vi "MonitorAlert.vi"(8 "error in (no error)":errorcluster, 10 "Str Refnum":refnum<vi>, 11 "Handle":i32) -> (0 "error out":errorcluster)   [LabVIEW 2016]
uses:
  kernel32.dll
panel:
  out "Array":u8[](array[numeric])
  out "Return":u8
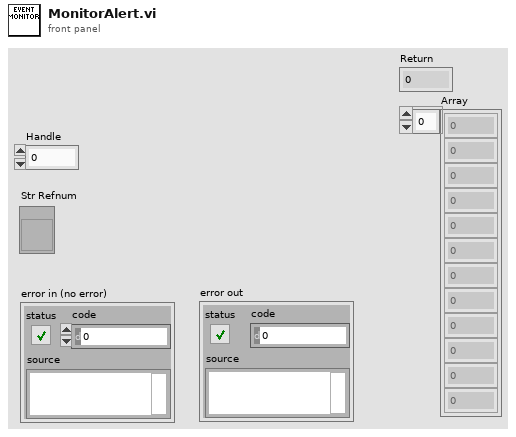
[diagram p1: front panel]
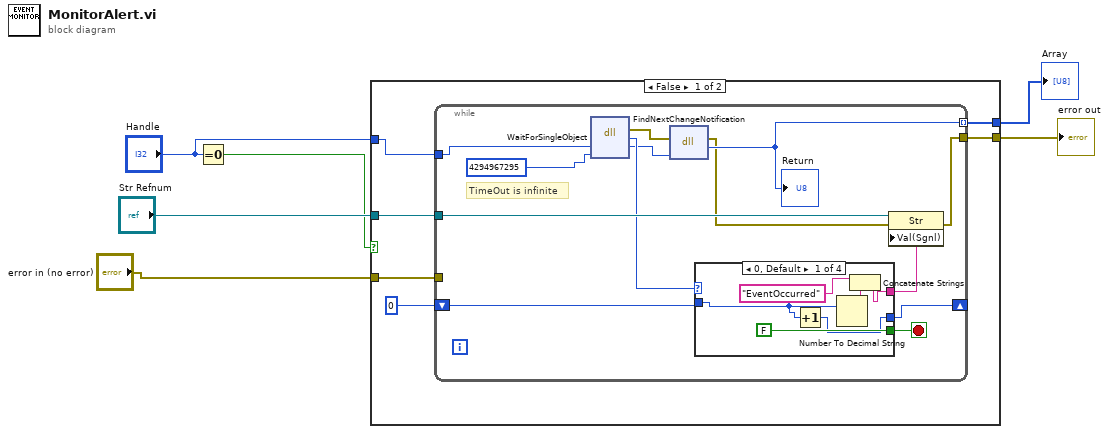
[diagram p0: block diagram]
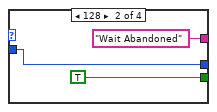
[diagram p2: hidden frame]
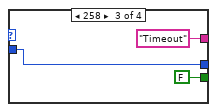
[diagram p3: hidden frame]
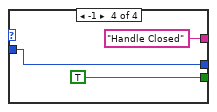
[diagram p4: hidden frame]
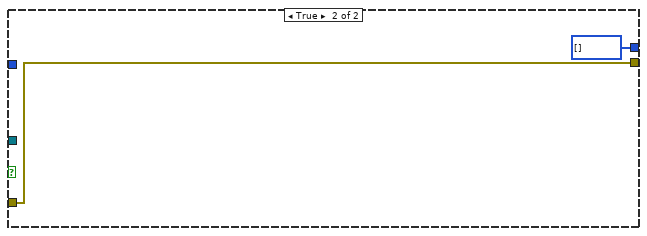
[diagram p5: hidden frame]
diagram:
  n1 = Equal To 0?(x="Handle") -> (x = 0?=w3:bool)
  n2 = case shown="False" w3 {
    tunnel: [w12 w42] -> w6
    tunnel: "Str Refnum" -> [w10 _]
    tunnel: "error in (no error)" -> [w9 w42]
    tunnel: "Handle" -> [w8 _]
    tunnel: [w7 u8[] []] -> w1
    frame False {
      n3 = while {
        tunnel: w8 -> [w21]
        tunnel: [w14] -> w12
        shift-right: [w24] -> _
        shift-left: 0 -> [w13]
        tunnel: w10 -> [w23]
        tunnel: w9 -> [_]
        tunnel: [w22] -> w7 mode=indexing
        stop <- w25 stop-if-true
        # "TimeOut is infinite"
        n4 = dll-call lib="kernel32.dll" fn="WaitForSingleObject"("Handle"=w21, "dwMilliseconds"=u32 4294967295) -> (error out=w16:errorcluster, "Return"=w19:u32, "Handle"=w18:i32)  [unwired: 4 in, 1 out]
        n5 = dll-call lib="kernel32.dll" fn="FindNextChangeNotification"(error in=w16, "Handle"=w18) -> (error out=w15:errorcluster, "Return"=w22:u8)  [unwired: 3 in, 1 out]
        "Return" <- w22
        n6 = case shown="0, Default" w19 {
          tunnel: [w28 "Wait Abandoned" ("String") "Timeout" ("String") "Handle Closed" ("String")] -> w17
          tunnel: [FALSE TRUE FALSE TRUE] -> w25
          tunnel: w13 -> [w27 w32 w35 w38]
          tunnel: [w26 w32 w35 w38] -> w24
          frame 0, Default {
            n7 = Increment(x=w27) -> (x+1=w26:i32)
            n8 = Number To Decimal String(number=w27) -> (decimal integer string=w29:string)  [unwired: 1 in]
            n9 = Concatenate Strings("EventOccurred" ("String"), w29) -> (w28:string)
          }
          frame 128 {
          }
          frame 258 {
          }
          frame -1 {
          }
        }
        n10 = property class="Str"(reference=w23, error in=w15, "Val(Sgnl)"=w17) -> (error out=w14:errorcluster)  [unwired: 1 out]
      }
    }
    frame True {
    }
  }
  "error out" <- w6
  "Array" <- w1
